vi "R1SBRControl_Manual.vi"(6 "ReleaseValve":bool, 7 "LabVIEW Web Service Request":refnum<class "Web Request.lvclass">, 8 "GasPump":bool, 9 "WaterPump":bool, 10 "EffluentPump":bool, 11 "MediaPump":bool) -> (3 "R1_SBR_Manual":T1)   [LabVIEW 2016]
uses:
  <vilib>/wsapi/Web Request.lvclass
panel:
  # "Use the Web Service Request input terminal to call the VIs on the Web Services palette. Do not remove it from the connector pane unless you don't need access to the palette."
  # "Each additional control wired to the connector pane will be available as an input in the URL. To include an indicator in terminal-mode output (the default setting), it must also be wired to the connector pane."
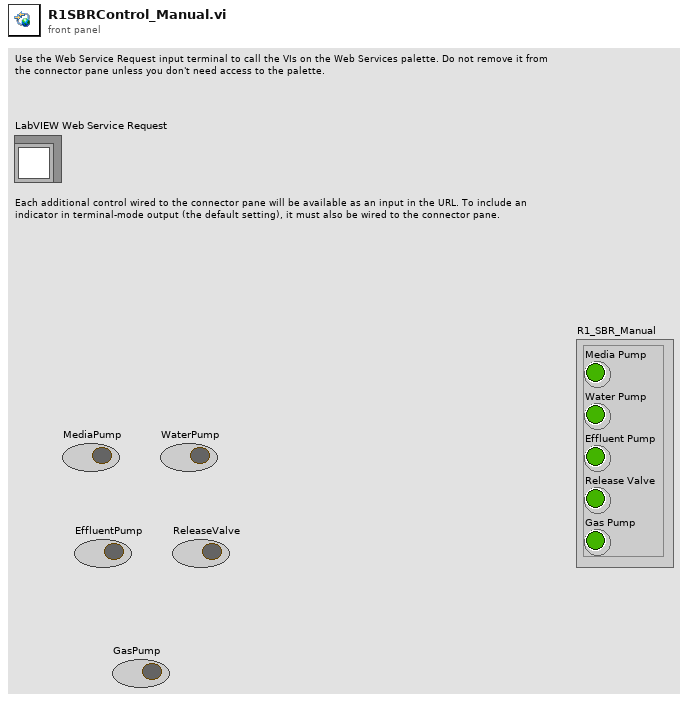
[diagram p1: front panel]
types:
  T1 = cluster{"Media Pump":bool, "Water Pump":bool, "Effluent Pump":bool, "Release Valve":bool, "Gas Pump":bool}
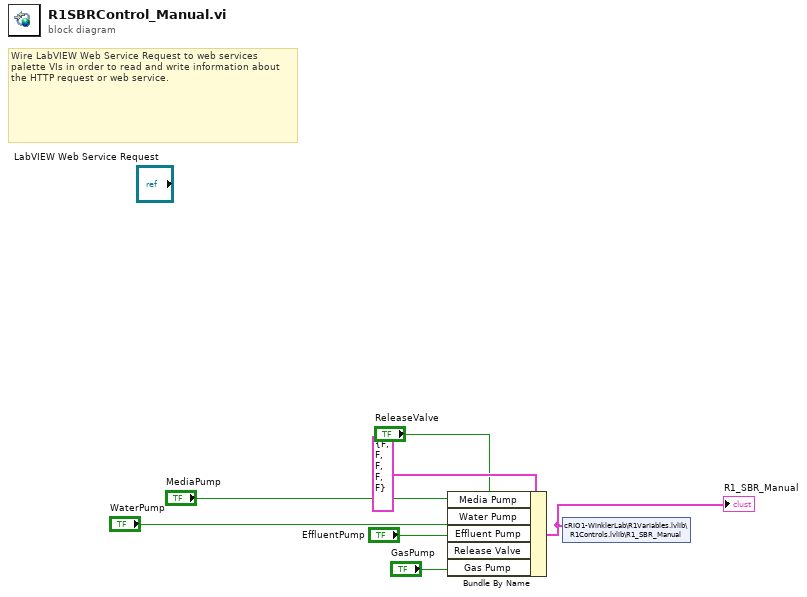
[diagram p0: block diagram]
diagram:
  # "Wire LabVIEW Web Service Request to web services palette VIs in order to read and write information about the HTTP request or web service."
  n1 = Bundle By Name(cluster=T1 {"Media Pump"=FALSE, "Water Pump"=FALSE, "Effluent Pump"=FALSE, "Release Valve"=FALSE, "Gas Pump"=FALSE} ("R1_SBR_Manual"), "Media Pump"="MediaPump", "Water Pump"="WaterPump", "Effluent Pump"="EffluentPump", "Release Valve"="ReleaseValve", "Gas Pump"="GasPump") -> (w6:T1)
  "R1_SBR_Manual" <- w6
  n2 = shared-variable "cRIO1-WinklerLab\\R1Variables.lvlib\\R1Controls.lvlib\\R1_SBR_Manual"(w6) -> ()  [unwired: 1 in, 1 out]
